vi "Open TLCamera.vi"(8 "error in (no error)":errorcluster, 9 "isDiagnosticsMessagesEnabled":bool, 10 "Camera serial number":string, 11 "TLCameraSDK reference":refnum<k24>) -> (0 "error out":errorcluster, 2 "TLCamera reference out":refnum<k24>, 3 "TLCameraSDK reference out":refnum<k24>)   [LabVIEW 2015]
uses:
  C:/code/Host/Installer/Scientific Camera Interfaces/LabVIEW/64_bit/Library_X64/Thorlabs.TSI.TLCameraInterfaces.dll
  64_bit/Library_X64/Thorlabs.TSI.TLCameraInterfaces.dll
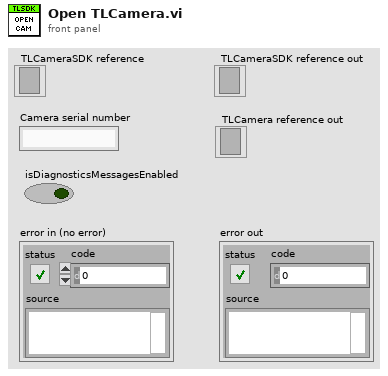
[diagram p1: front panel]
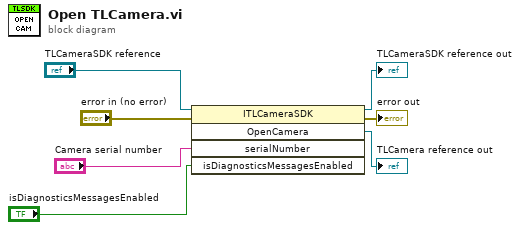
[diagram p0: block diagram]
diagram:
  n1 = invoke class="ITLCameraSDK" method="OpenCamera"(reference="TLCameraSDK reference", error in="error in (no error)", "serialNumber"="Camera serial number", "isDiagnosticsMessagesEnabled"="isDiagnosticsMessagesEnabled") -> (reference out=→"TLCameraSDK reference out":refnum<k24>, error out=→"error out":errorcluster, "OpenCamera"=→"TLCamera reference out":refnum<k24>)  [unwired: 1 in, 2 out]
